vi "Destructor.vi"(8 "Error In":errorcluster, 11 "Spaceship in":refnum<class "Spaceship.lvclass">) -> (0 "Error Out":errorcluster, 3 "Spaceship out":refnum<class "Spaceship.lvclass">)   [LabVIEW 2021, in "Spaceship.lvclass"]
doc: "Relase queue in class object."
uses:
  Spaceship.lvclass
  Spaceship.lvclass/Spaceship.ctl
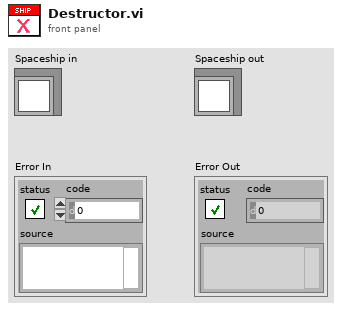
[diagram p1: front panel]
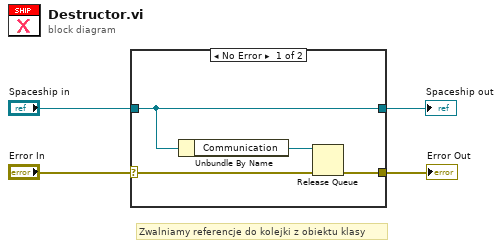
[diagram p0: block diagram]
diagram:
  # "Zwalniamy referencje do kolejki z obiektu klasy"
  n1 = case shown="No Error" "Error In" {
    selector: "Error In" -> [w6 w10]
    tunnel: [w5 w10] -> w3
    tunnel: [w8 w9] -> w1
    tunnel: "Spaceship in" -> [w8 w9]
    frame No Error {
      n2 = Unbundle By Name(w8) -> ("Communication"=w7:refnum<queue>)
      n3 = Release Queue(queue=w7, error in (no error)=w6) -> (error out=w5:errorcluster)  [unwired: 1 in, 2 out]
    }
    frame Error {
    }
  }
  "Error Out" <- w3
  "Spaceship out" <- w1
